vi "Stop Core.vi"(10 "final error code":i32, 11 "Master Controller in":refnum<class "Master Controller.lvclass">) -> (3 "Master Controller out":refnum<class "Master Controller.lvclass">)   [LabVIEW 2015, in "Master Controller Core.lvlib" / "Master Controller.lvclass"]
doc: "(<B>Filename</B>: Actor Framework.lvlib:Actor.lvclass:Stop Core.vi)\n\nDefines what the actor does before it stops. Use the <B>final error code</B> input to determine whether the actor shut down in response to an error.\n\nBy default, this method does nothing. A descendant class may override it to define behavior, such as shutting down any processes the actor initiated in its override of the Actor Core method."
uses:
  Master Controller.lvclass
  Utilities/Status Messaging.llb/Status Message Command.ctl
  Master Controller.lvclass/Master Controller.ctl
  <vilib>/ActorFramework/Message Enqueuer/Message Enqueuer.lvclass/Message Enqueuer.ctl
  <vilib>/ActorFramework/Message Enqueuer/Enqueue.vi
  <vilib>/ActorFramework/Message Priority Queue/Priority Enqueue.vi
  <vilib>/ActorFramework/Actor/Actor.lvclass
  <vilib>/ActorFramework/Stop Msg/Stop Msg.lvclass
  Utilities/Status Messaging.llb/Status Messaging.lvlib
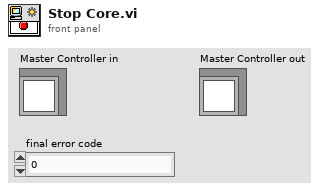
[diagram p1: front panel]
types:
  T1 = typedef "Status Messaging.lvlib/Status Message Command.ctl" = enum16{"Write", "Obtain", "Kill"}
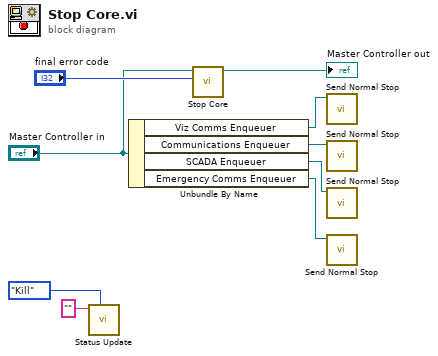
[diagram p0: block diagram]
diagram:
  n1 = call "Status Update.vi"("Command (Write)"=Status_Message_Command."Kill", "Status Update"="") -> ()  [unwired: 8 in, 2 out]
  n2 = Unbundle By Name("Master Controller in") -> ("Viz Comms Enqueuer"=w1:refnum<class "Message Enqueuer.lvclass">, "Communications Enqueuer"=w4:refnum<class "Message Enqueuer.lvclass">, "SCADA Enqueuer"=w5:refnum<class "Message Enqueuer.lvclass">, "Emergency Comms Enqueuer"=w6:refnum<class "Message Enqueuer.lvclass">)
  n3 = call-parent "Stop Core.vi"("final error code"="final error code", "Actor in"="Master Controller in") -> ("Actor out"=→"Master Controller out":refnum<class "Master Controller.lvclass">)  [unwired: 9 in]
  n4 = call <vilib>:"Send Normal Stop.vi"("Message Enqueuer"=w1) -> ()  [unwired: 10 in, 1 out]
  n5 = call <vilib>:"Send Normal Stop.vi"("Message Enqueuer"=w4) -> ()  [unwired: 10 in, 1 out]
  n6 = call <vilib>:"Send Normal Stop.vi"("Message Enqueuer"=w5) -> ()  [unwired: 10 in, 1 out]
  n7 = call <vilib>:"Send Normal Stop.vi"("Message Enqueuer"=w6) -> ()  [unwired: 10 in, 1 out]
